vi "Find-str-in-string-array.vi"(10 "str array":string[](array[string]), 11 "str":string) -> (2 "found index":i32)   [LabVIEW 2020]
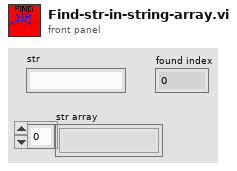
[diagram p1: front panel]
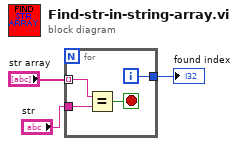
[diagram p0: block diagram]
diagram:
  n1 = for {
    tunnel: "str array" -> [w6] mode=indexing
    tunnel: "str" -> [w7]
    tunnel: [w4] -> w1
    i -> [w4]
    stop <- w5 stop-if-true
    n2 = Equal?(x=w6, y=w7) -> (x = y?=w5:bool)
  }
  "found index" <- w1
